vi "RichToFlatnixnet_grpc_ConvertTimestamp1nsTo100nsRequest.vi"(5 "OutputClusterType":T1, 11 "InputCluster":T2) -> (3 "OutputCluster":T1)   [LabVIEW 2025, in "grpc-xnet_client.lvlib"]
uses:
  grpc-xnet_client.lvlib
  nixnet_grpc_ConvertTimestamp1nsTo100nsRequest.ctl
  nixnet_grpc_ConvertTimestamp1nsTo100nsRequest_Flat.ctl
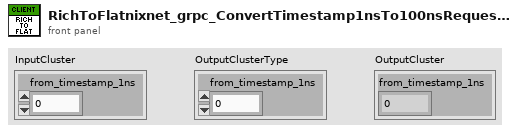
[diagram p1: front panel]
types:
  T1 = typedef "grpc-xnet_client.lvlib/nixnet_grpc_ConvertTimestamp1nsTo100nsRequest_Flat.ctl" = cluster{"from_timestamp_1ns":u64}
  T2 = typedef "grpc-xnet_client.lvlib/nixnet_grpc_ConvertTimestamp1nsTo100nsRequest.ctl" = cluster{"from_timestamp_1ns":u64}
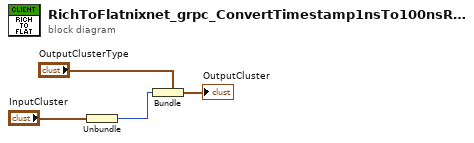
[diagram p0: block diagram]
diagram:
  n1 = Unbundle "Unbundle"("InputCluster") -> ("from_timestamp_1ns"=w1:u64)
  n2 = Bundle "Bundle"(cluster="OutputClusterType", "from_timestamp_1ns"=w1) -> (→"OutputCluster":T1)
